vi "Aircraft Discovery Main.vi"(7 "Aircraft ID":u8, 8 "Error In":errorcluster, 11 "MavLINK Message":string) -> (0 "Error Out":errorcluster)   [LabVIEW 2014]
uses:
  Controls/Aircraft Discovery State.ctl
  Controls/Known Aircraft.ctl
  Hardware Driver/Controls/Coms Driver Interface.ctl
  Telemetry/Controls/Telemetry Connection Type.ctl
  Overlord/SubVI/Message Queues/Tx to Overlord/SubVI/Send MAVLink to Overlord.vi
  SubVI/Queue References/SubVI/Get Aircraft RX Queue String.vi
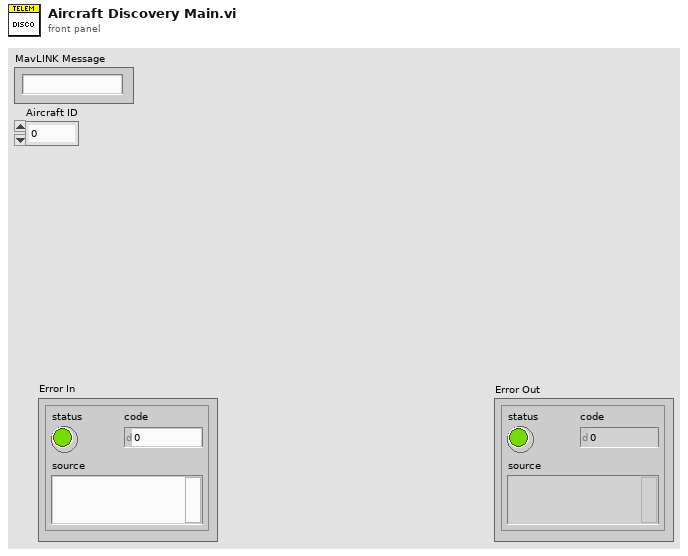
[diagram p1: front panel]
types:
  T1 = typedef "Aircraft Discovery State.ctl" = enum16{"Initalise", "Check If Known Aircraft", "Route to known coms instance", "Create coms instance for new aircraft", "Complete"}
  T2 = typedef "Known Aircraft.ctl" = cluster{"Aircraft ID":u8, "Aircraft Receive queue Ref":refnum<queue>, "Aircraft Transmit queue Ref":refnum<queue>, "Waypoint Queue Ref":refnum<queue>, "Connection Details":T3}
  T3 = typedef "Coms Driver Interface.ctl" = cluster{"Connection Type":T4, "UDP connection ID":refnum<k16>, "Serial COM port ID":refnum<visa-resource-name>, "IP Address of Aircraft":u32}
  T4 = typedef "Telemetry Connection Type.ctl" = enum16{"Serial", "UDP", "TCP"}
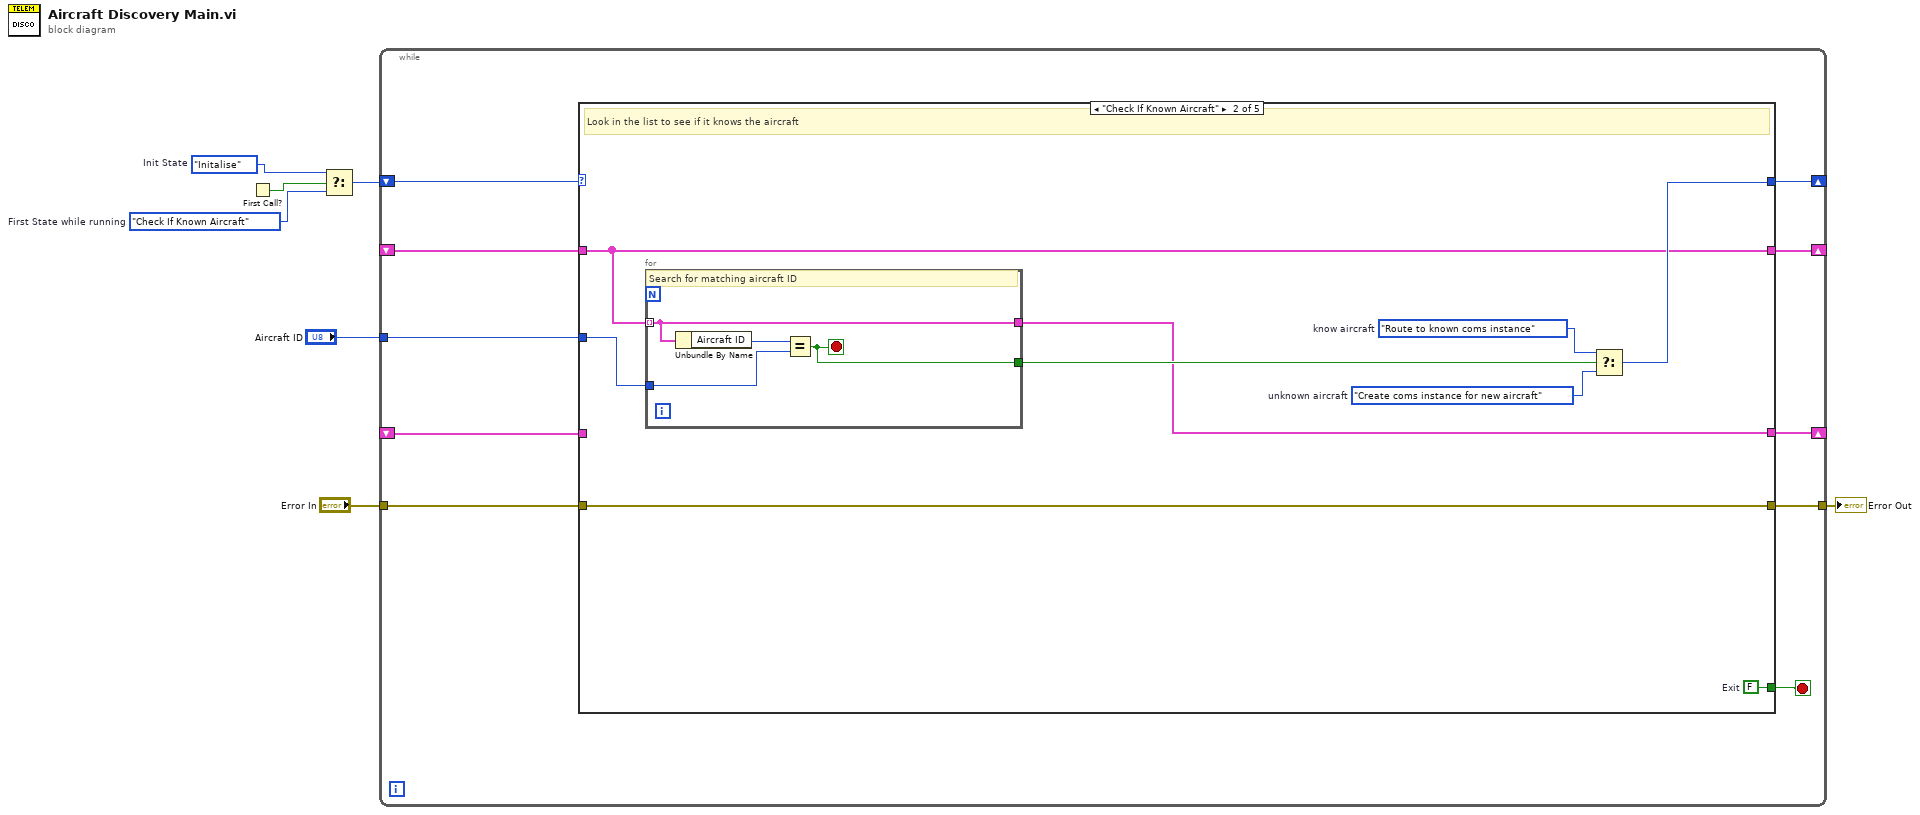
[diagram p0: block diagram]
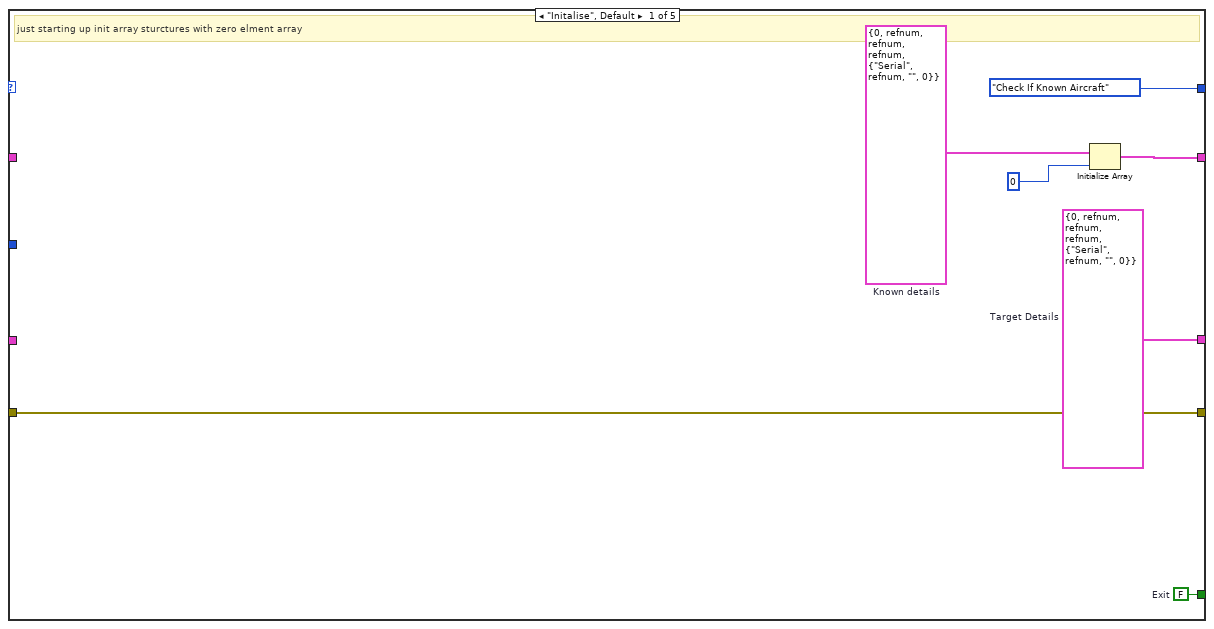
[diagram p2: hidden frame]
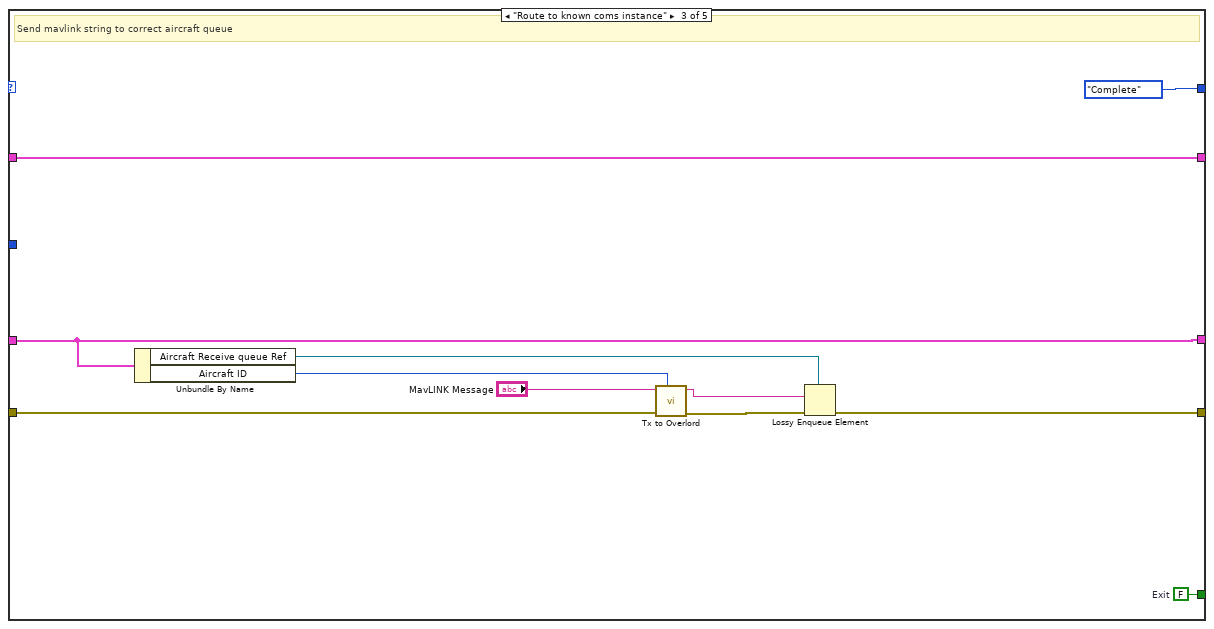
[diagram p3: hidden frame]
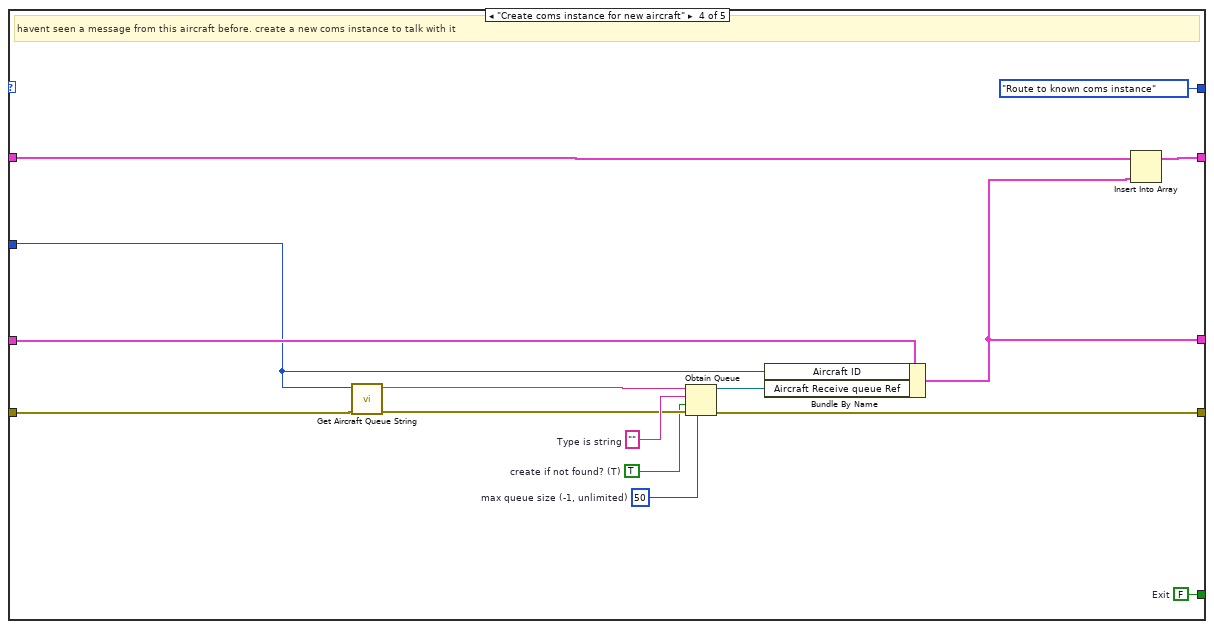
[diagram p4: hidden frame]
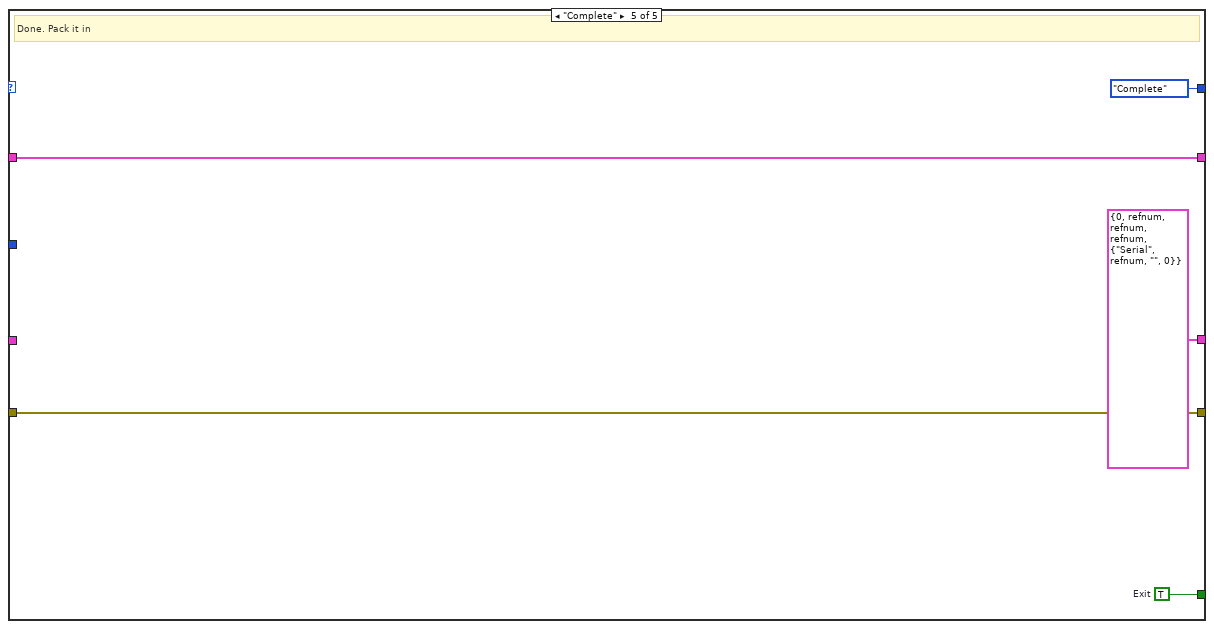
[diagram p5: hidden frame]
diagram:
  w5 = Aircraft_Discovery_State."Check If Known Aircraft"  # First State while running
  w6 = Aircraft_Discovery_State."Initalise"  # Init State
  n1 = First Call?() -> (First Call?: T/F=w1:bool)
  n2 = Select(t=w6, s=w1, f=w5) -> (s? t:f=w4:T1)
  n3 = while {
    tunnel: "Aircraft ID" -> [w17]
    shift-right: [w15] -> _
    shift-left: w4 -> [w16]
    tunnel: "Error In" -> [w14]
    tunnel: [w13] -> w2
    shift-right: [w12] -> _
    shift-left: _ -> [w11]
    shift-right: [w10] -> _
    shift-left: _ -> [w9]
    stop <- w8 stop-if-true
    n4 = case shown="\"Check If Known Aircraft\"" w16 {
      tunnel: w17 -> [_ w28 _ w49 _]
      tunnel: [Aircraft_Discovery_State."Check If Known Aircraft" ("First State while running") w31 Aircraft_Discovery_State."Complete" ("unknown aircraft") Aircraft_Discovery_State."Route to known coms instance" ("unknown aircraft") Aircraft_Discovery_State."Complete" ("unknown aircraft")] -> w15
      tunnel: w14 -> [w23 w30 w43 w57 w64]
      tunnel: [w23 w30 w42 w53 w64] -> w13
      tunnel: [w22 w29 w46 w58 w67] -> w12
      tunnel: w11 -> [_ w29 w46 w59 w67]
      tunnel: [w19 w26 w39 w52 T2 {"Aircraft ID"=0, "Aircraft Receive queue Ref"=refnum, "Aircraft Transmit queue Ref"=refnum, "Waypoint Queue Ref"=refnum, "Connection Details"={"Connection Type"=enum."Serial", "UDP connection ID"=refnum, "Serial COM port ID"="", "IP Address of Aircraft"=0}} ("Target Details")] -> w10
      tunnel: w9 -> [_ _ w39 w55 _]
      tunnel: [w18 w25 w38 w50 w66] -> w8
      frame "Initalise", Default {
        w18 = FALSE  # Exit
        w19 = T2 {"Aircraft ID"=0, "Aircraft Receive queue Ref"=refnum, "Aircraft Transmit queue Ref"=refnum, "Waypoint Queue Ref"=refnum, "Connection Details"={"Connection Type"=enum."Serial", "UDP connection ID"=refnum, "Serial COM port ID"="", "IP Address of Aircraft"=0}}  # Target Details
        w21 = T2 {"Aircraft ID"=0, "Aircraft Receive queue Ref"=refnum, "Aircraft Transmit queue Ref"=refnum, "Waypoint Queue Ref"=refnum, "Connection Details"={"Connection Type"=enum."Serial", "UDP connection ID"=refnum, "Serial COM port ID"="", "IP Address of Aircraft"=0}}  # Known details
        # "just starting up init array sturctures with zero elment array"
        n5 = Initialize Array(w21, 0 ("Known Aircraft ID")) -> (w22:T2[])
      }
      frame "Check If Known Aircraft" {
        w25 = FALSE  # Exit
        w32 = Aircraft_Discovery_State."Create coms instance for new aircraft"  # unknown aircraft
        w33 = Aircraft_Discovery_State."Route to known coms instance"  # know aircraft
        # "Look in the list to see if it knows the aircraft"
        n6 = for {
          tunnel: w29 -> [w34] mode=indexing
          tunnel: w28 -> [w36]
          tunnel: [w35] -> w27
          tunnel: [w34] -> w26
          stop <- w35 stop-if-true
          # "Search for matching aircraft ID"
          n7 = Unbundle By Name(w34) -> ("Aircraft ID"=w37:u8)
          n8 = Equal?(x=w37, y=w36) -> (x = y?=w35:bool)
        }
        n9 = Select(t=w33, s=w27, f=w32) -> (s? t:f=w31:T1)
      }
      frame "Route to known coms instance" {
        w38 = FALSE  # Exit
        # "Send mavlink string to correct aircraft queue"
        n10 = Unbundle By Name(w39) -> ("Aircraft Receive queue Ref"=w41:refnum<queue>, "Aircraft ID"=w44:u8)
        n11 = call-poly "Tx to Overlord.vi"("Aircraft ID"=w44, "Error In"=w43, "MAVLink String"="MavLINK Message") -> ("error out"=w48:errorcluster, "MAVLink String Out"=w40:string)  [unwired: 7 in]
        n12 = Lossy Enqueue Element(queue=w41, element=w40, error in (no error)=w48) -> (error out=w42:errorcluster)  [unwired: 3 out]
      }
      frame "Create coms instance for new aircraft" {
        w50 = FALSE  # Exit
        w51 = TRUE  # create if not found? (T)
        w60 = 50  # max queue size (-1, unlimited)
        w62 = ""  # Type is string
        # "havent seen a message from this aircraft before. create a new coms instance to talk with it"
        n13 = call-poly "Get Aircraft Queue String.vi"("Error In"=w57, "Aircraft ID"=w49) -> ("Error Out"=w56:errorcluster, "Aircraft Q Name"=w61:string)  [unwired: 8 in]
        n14 = Obtain Queue(max queue size (-1, unlimited)=w60, name (unnamed)=w61, element data type=w62, create if not found? (T)=w51, error in (no error)=w56) -> (queue out=w54:refnum<queue>, error out=w53:errorcluster)  [unwired: 1 out]
        n15 = Bundle By Name(cluster=w55, "Aircraft ID"=w49, "Aircraft Receive queue Ref"=w54) -> (w52:T2)
        n16 = Insert Into Array(array=w59, new element=w52) -> (w58:T2[])  [unwired: 1 in]
      }
      frame "Complete" {
        w66 = TRUE  # Exit
        # "Done. Pack it in"
      }
    }
  }
  "Error Out" <- w2
